vi "SPUR_RANGE_ENABLE.vi"(0 "Session In":refnum<visa-resource-name>="TCPIP0::K-N90X0A-00005.local::inst0::INSTR", 2 "Timeout":u32=3000, 5 "error in":errorcluster {"code" format="%.0x"}, 6 "ALL Ranges OFF":bool, 7 "WRITE":bool, 9 "READ":bool, 11 "Range#":i32, 13 "ON/OFF":bool) -> (14 "Session Out":refnum<visa-resource-name>, 19 "error out":errorcluster {"code" format="%.0x"})   [LabVIEW 2018]
doc: "Launches the Instrument I/O Assistant, which you can use to communicate with message-based instruments and graphically parse the response. For example you can communicate with an instrument that uses a serial, Ethernet, or GPIB interface."
panel:
  in  "ALL Ranges ON":bool
  out "spreadsheet string":string
  out "output array":dbl[](array[numeric])
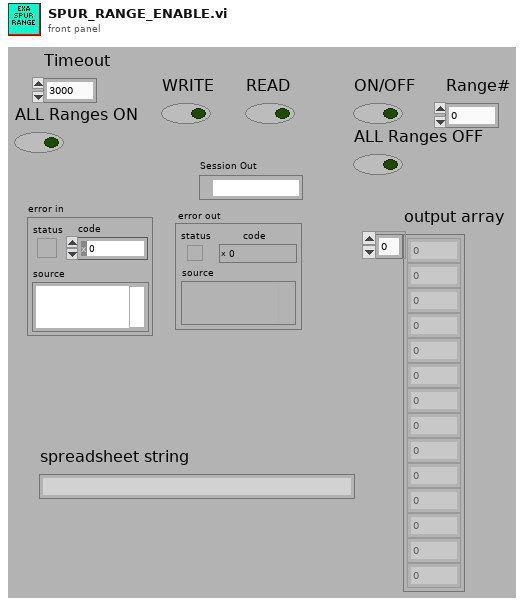
[diagram p1: front panel]
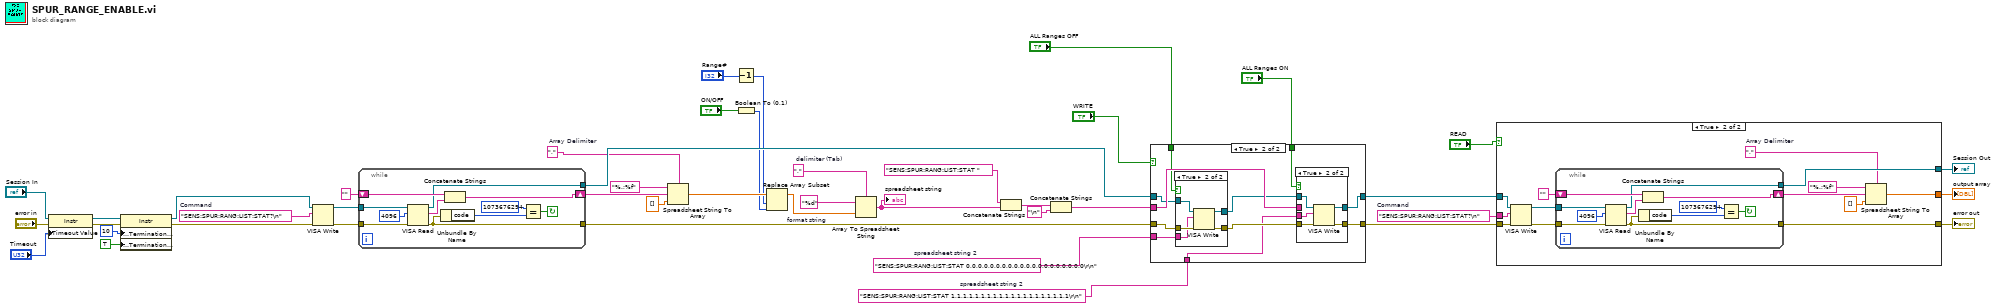
[diagram p0: block diagram]
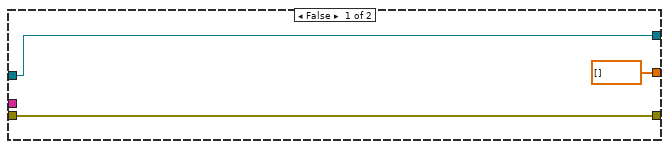
[diagram p2: hidden frame]
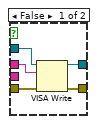
[diagram p5: hidden frame]
diagram:
  w3 = "SENS:SPUR:RANG:LIST:STAT 1,1,1,1,1,1,1,1,1,1,1,1,1,1,1,1,1,1,1,1\r\n"  # spreadsheet string 2
  w5 = ","  # Array Delimiter
  w12 = "SENS:SPUR:RANG:LIST:STAT 0,0,0,0,0,0,0,0,0,0,0,0,0,0,0,0,0,0,0,0\r\n"  # spreadsheet string 2
  w17 = "SENS:SPUR:RANG:LIST:STAT?\n"  # Command
  w24 = "%d"  # format string
  w25 = ","  # delimiter (Tab)
  w34 = "SENS:SPUR:RANG:LIST:STAT?\n"  # Command
  n1 = property class="Instr"(reference="Session In", error in="error in", "General Settings:Timeout Value"="Timeout") -> (reference out=w39:refnum<visa-resource-name>, error out=w41:errorcluster)
  n2 = property class="Instr"(reference=w39, error in=w41, "Message Based Settings:Termination Character"=u8 10 ("Termination Char"), "Message Based Settings:Termination Character Enable"=TRUE ("enable")) -> (reference out=w31:refnum<visa-resource-name>, error out=w32:errorcluster)
  n3 = VISA Write(VISA resource name=w31, write buffer=w34, error in (no error)=w32) -> (VISA resource name out=w11:refnum<visa-resource-name>, error out=w10:errorcluster)  [unwired: 1 out]
  n4 = while {
    tunnel: w11 -> [w52]
    shift-right: [w46] -> w6
    shift-left: "" -> [w51]
    tunnel: w10 -> [w49]
    tunnel: [w48] -> w30
    tunnel: [w45] -> w29
    stop <- w47 continue-if-true
    n5 = VISA Read(VISA resource name=w52, byte count=u32 4096 ("byte count (0)"), error in (no error)=w49) -> (VISA resource name out=w45:refnum<visa-resource-name>, read buffer=w50:string, error out=w48:errorcluster)  [unwired: 1 out]
    n6 = Unbundle By Name(w48) -> ("code"=w54:i32)
    n7 = Concatenate Strings(w51, w50) -> (w46:string)
    n8 = Equal?(x=1073676294, y=w54) -> (x = y?=w47:bool)
  }
  n9 = Spreadsheet String To Array(delimiter (Tab)=w5, format string="%.;%f", spreadsheet string=w6, array type (2D Dbl)=dbl[] []) -> (array=w28:dbl[])
  n10 = Decrement(x="Range#") -> (x-1=w22:i32)
  n11 = Boolean To (0,1)(Boolean="ON/OFF") -> (0, 1=w13:i16)
  n12 = Replace Array Subset(array=w28, new element=w13, index=w22) -> (w26:dbl[])
  n13 = Array To Spreadsheet String(delimiter (Tab)=w25, array=w26, 3:w24) -> (spreadsheet string=w23:string)
  "spreadsheet string" <- w23
  n14 = Concatenate Strings("SENS:SPUR:RANG:LIST:STAT " ("staticText"), w23) -> (w36:string)
  n15 = Concatenate Strings(w36, "\n" ("StaticText")) -> (w27:string)
  n16 = case shown="True" "WRITE" {
    tunnel: w30 -> [w57 w65]
    tunnel: [w57 w68] -> w20
    tunnel: w29 -> [w56 w60]
    tunnel: [w56 w67] -> w21
    tunnel: w27 -> [_ w66]
    tunnel: w12 -> [_ w58]
    tunnel: "ALL Ranges OFF" -> [_ w62]
    tunnel: "ALL Ranges ON" -> [_ w61]
    tunnel: w3 -> [_ w59]
    frame False {
    }
    frame True {
      n17 = case shown="True" w62 {
        tunnel: w65 -> [w69 w75]
        tunnel: [w69 w74] -> w64
        tunnel: w60 -> [w70 w72]
        tunnel: [w70 w73] -> w63
        tunnel: w58 -> [_ w71]
        frame False {
        }
        frame True {
          n18 = VISA Write(VISA resource name=w72, write buffer=w71, error in (no error)=w75) -> (VISA resource name out=w73:refnum<visa-resource-name>, error out=w74:errorcluster)  [unwired: 1 out]
        }
      }
      n19 = case shown="True" w61 {
        tunnel: w64 -> [w80 w85]
        tunnel: [w79 w84] -> w68
        tunnel: w63 -> [w78 w83]
        tunnel: [w77 w82] -> w67
        tunnel: w66 -> [w76 _]
        tunnel: w59 -> [_ w81]
        frame False {
          n20 = VISA Write(VISA resource name=w78, write buffer=w76, error in (no error)=w80) -> (VISA resource name out=w77:refnum<visa-resource-name>, error out=w79:errorcluster)  [unwired: 1 out]
        }
        frame True {
          n21 = VISA Write(VISA resource name=w83, write buffer=w81, error in (no error)=w85) -> (VISA resource name out=w82:refnum<visa-resource-name>, error out=w84:errorcluster)  [unwired: 1 out]
        }
      }
    }
  }
  n22 = case shown="True" "READ" {
    tunnel: w20 -> [w86 w101]
    tunnel: w17 -> [_ w97]
    tunnel: [dbl[] [] w93] -> w15
    tunnel: [w87 w92] -> w18
    tunnel: w21 -> [w87 w91]
    tunnel: [w86 w89] -> w19
    frame False {
    }
    frame True {
      w90 = ","  # Array Delimiter
      n23 = VISA Write(VISA resource name=w91, write buffer=w97, error in (no error)=w101) -> (VISA resource name out=w100:refnum<visa-resource-name>, error out=w99:errorcluster)  [unwired: 1 out]
      n24 = while {
        tunnel: w100 -> [w109]
        shift-right: [w103] -> w94
        shift-left: "" -> [w108]
        tunnel: w99 -> [w106]
        tunnel: [w105] -> w89
        tunnel: [w102] -> w92
        stop <- w104 continue-if-true
        n25 = VISA Read(VISA resource name=w109, byte count=u32 4096 ("byte count (0)"), error in (no error)=w106) -> (VISA resource name out=w102:refnum<visa-resource-name>, read buffer=w107:string, error out=w105:errorcluster)  [unwired: 1 out]
        n26 = Unbundle By Name(w105) -> ("code"=w111:i32)
        n27 = Concatenate Strings(w108, w107) -> (w103:string)
        n28 = Equal?(x=1073676294, y=w111) -> (x = y?=w104:bool)
      }
      n29 = Spreadsheet String To Array(delimiter (Tab)=w90, format string="%.;%f", spreadsheet string=w94, array type (2D Dbl)=dbl[] []) -> (array=w93:dbl[])
    }
  }
  "Session Out" <- w18
  "error out" <- w19
  "output array" <- w15
